vi "HB_ImaqLLGrab.vi"() -> ()   [LabVIEW 2009, in "HB_IMAQ_Examples.lvlib"]
doc: "The HL Grab VI acquires images continuously and displays the images in an image control using high-level acquisition VIs. A grab is appropriate for high-speed applications that process only one image at a time.\n\nIMAQ Init initializes the device. IMAQ Grab Setup initializes the grab function and starts capturing images to an internal software buffer. IMAQ Create creates an image buffer. IMAQ Grab Acquire copies the internal buffer to Image out, and an image control displays the image on the front panel. IMAQ Close releases resources associated with the acquisition, and IMAQ Dispose frees the image buffer."
uses:
  <vilib>/vision/driver/IMAQdx.llb/IMAQdx Buffer Number Mode.ctl
  lib.lib/HGF_LVC/HGF_IMAQ/HGF_IMAQFactory/HGF_IMAQFactory.lvclass
  lib.lib/HGF_LVC/HGF_IMAQ/HGF_IMAQDevice/HGF_IMAQDevice.lvclass
  HB_IMAQ_Examples.lvlib
  lib.lib/HGF_LVC/HGF_BaseClasses/HGF_Factory/HGF_Factory.lvclass
  lib.lib/HGF_LVC/HGF_DeviceBaseClasses/HGF_DeviceBase/HGF_DeviceBase.lvclass
  lib.lib/HGF_LVC/HGF_Auxiliary/HGF_Auxiliary.lvlib
  lib.lib/VisionTools/HGF_VisionTools/HGF_VisionTools.lvlib
  <vilib>/vision/driver/NI_Vision_Acquisition_Software.lvlib
panel:
  in  "Buffer Number Mode (Next)":T1
  out "error out":errorcluster
  in  "Number of buffers":u32=2
  out "processed FPS":dbl
  out "acquired FPS":dbl
  out "iteration":i32
  out "Image":T2(plugin-control)
  in  "interval / ms":u32=100
  in  "stop":bool
  in  "Image Type":T3 items=["Grayscale (U8)", "Grayscale (I16)", "Grayscale (SGL)", "Complex (CSG)", "RGB (U32)", "HSL (U32)", "RGB (U64)", "Grayscale (U16)"]
  in  "cameraName":string="cam0"
  in  "imaqClassName":string="HGF_ImaqDx"
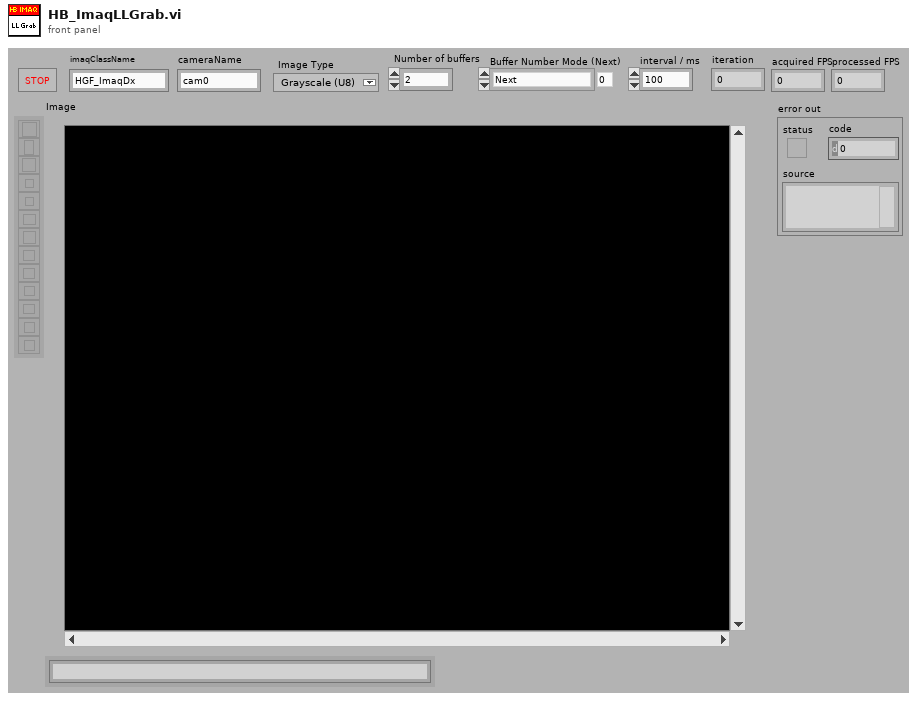
[diagram p1: front panel]
types:
  T1 = typedef "NI_Vision_Acquisition_Software.lvlib/IMAQdx Buffer Number Mode.ctl" = enum32{"Next", "Last", "Buffer Number"}
  T2 = typedef "IMAQ Image.ctl" = refnum<image>
  T3 = typedef "Image Type" = u32
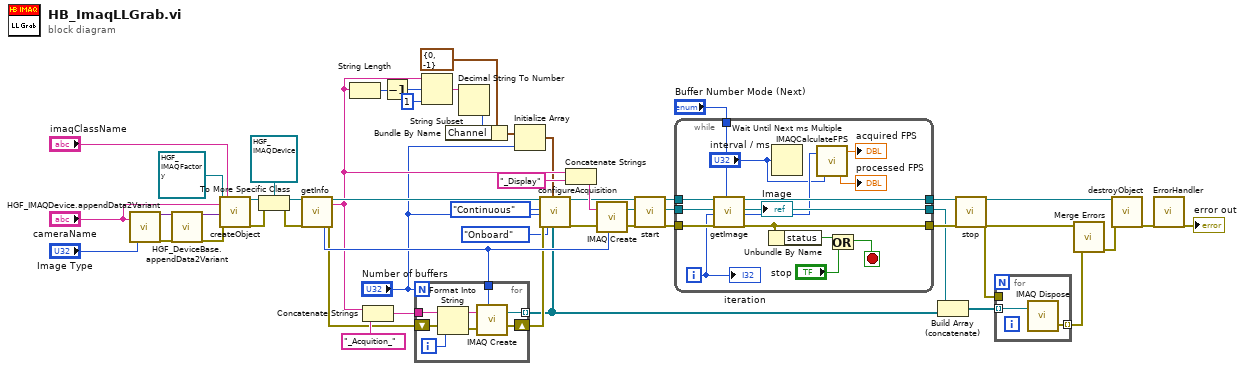
[diagram p0: block diagram]
diagram:
  n1 = call "HGF_IMAQDevice.appendData2Variant.vi"("cameraName"="cameraName", "imageType"="Image Type") -> ("dup initData"=w51:variant, "error out"=w50:errorcluster)  [unwired: 4 in, 12 out]
  n2 = call "HGF_DeviceBase.appendData2Variant.vi"("initData"=w51, "error in (no error)"=w50) -> ("dup initData"=w48:variant, "error out"=w49:errorcluster)  [unwired: 16 out]
  n3 = call "createObject.vi"("HGF_Factory"=refnum<class "HGF_IMAQFactory.lvclass"> refnum ("HGF_IMAQ.lvlib:HGF_IMAQFactory.lvclass"), "objectName"="cameraName", "initializationData"=w48, "error in (no error)"=w49, "className"="imaqClassName") -> ("HGF_Object"=w46:refnum<class "HGF_Factory.lvclass">, "error out"=w45:errorcluster)  [unwired: 13 out]
  n4 = To More Specific Class(target class=refnum<class "HGF_IMAQDevice.lvclass"> refnum ("HGF_DeviceBaseClasses.lvlib:HGF_IMAQDevice.lvclass"), reference=w46, error in=w45) -> (specific class reference=w42:refnum<class "HGF_IMAQDevice.lvclass">, error out=w41:errorcluster)
  n5 = call "getInfo.vi"("HGF_IMAQDevice"=w42, "error in (no error)"=w41) -> ("imageType"=w36:T3, "dup HGF_IMAQDevice"=w30:refnum<class "HGF_IMAQDevice.lvclass">, "cameraName"=w12:string, "error out"=w28:errorcluster)  [unwired: 12 in, 2 out]
  n6 = String Length(string=w12) -> (length=w11:i32)
  n7 = Concatenate Strings(w12, "_Acquition_" ("string")) -> (w29:string)
  n8 = Decrement(x=w11) -> (x-1=w10:i32)
  n9 = for {
    N: "Number of buffers" -> [_]
    tunnel: w36 -> [w59]
    tunnel: w29 -> [w57]
    shift-right: [w58] -> w35
    shift-left: w28 -> [w55]
    tunnel: [w52] -> w22 mode=indexing
    i -> [w53]
    n10 = Format Into String(initial string=w57, error in=w55, w53) -> (resulting string=w56:string, error out=w54:errorcluster)  [unwired: 1 in]
    n11 = call "IMAQ Create"("Image Name"=w56, "Image Type"=w59, "error in (no error)"=w54) -> ("New Image"=w52:T2, "error out"=w58:errorcluster)  [unwired: 1 in, 1 out]
  }
  n12 = String Subset(string=w12, offset (0)=w10, length (rest)=1 ("length (rest)")) -> (substring=w7:string)
  n13 = Decimal String To Number(string=w7) -> (number=w6:i32)  [unwired: 3 out]
  n14 = Bundle By Name(cluster=cluster{"Skip Count":u32, "Channel":i32} {"Skip Count"=0, "Channel"=-1} ("Buffer Parameter"), "Channel"=w6) -> (w5:cluster{"Skip Count":u32, "Channel":i32})
  n15 = Initialize Array(w5, "Number of buffers") -> (w3:cluster{"Skip Count":u32, "Channel":i32}[])
  n16 = call "configureAcquisition.vi"("HGF_IMAQDevice"=w30, "Continuous?"=enum16{"One-Shot", "Continuous"}."Continuous", "Number of buffers"="Number of buffers", "error in (no error)"=w35, "Memory Location"=enum16{"System", "Onboard"}."Onboard", "Buffer Parameters"=w3, "Image Array"=w22) -> ("dup HGF_IMAQDevice"=w27:refnum<class "HGF_IMAQDevice.lvclass">, "error out"=w34:errorcluster)  [unwired: 11 in]
  n17 = Concatenate Strings(w12, "_Display" ("string")) -> (w38:string)
  n18 = call "IMAQ Create"("Image Name"=w38, "Image Type"=w36, "error in (no error)"=w34) -> ("New Image"=w23:T2, "error out"=w25:errorcluster)  [unwired: 1 in, 1 out]
  n19 = call "start.vi"("HGF_IMAQDevice"=w27, "error in (no error)"=w25) -> ("dup HGF_IMAQDevice"=w26:refnum<class "HGF_IMAQDevice.lvclass">, "error out"=w24:errorcluster)  [unwired: 16 in]
  n20 = while {
    tunnel: w26 -> [w71]
    tunnel: w24 -> [w70]
    tunnel: w23 -> [w67]
    tunnel: [w66] -> w18
    tunnel: [w69] -> w19
    tunnel: [w68] -> w21
    tunnel: "Buffer Number Mode (Next)" -> [w64]
    i -> [w65]
    stop <- w72 stop-if-true
    n21 = call "getImage.vi"("HGF_IMAQDevice"=w71, "Image In"=w67, "Buffer Number"=w65, "error in (no error)"=w70, "Buffer Number Mode (Next)"=w64) -> ("dup HGF_IMAQDevice"=w68:refnum<class "HGF_IMAQDevice.lvclass">, "Image Out"=w66:T2, "Buffer Number Copied"=w63:i32, "error out"=w69:errorcluster)  [unwired: 8 in, 3 out]
    "Image" <- w66
    n22 = Unbundle By Name(w69) -> ("status"=w74:bool)
    n23 = Wait Until Next ms Multiple(millisecond multiple="interval / ms") -> ()  [unwired: 1 out]
    n24 = call "IMAQCalculateFPS.vi"("Update interval"="interval / ms", "buffer number"=w63) -> ("processed FPS"=→"processed FPS":dbl, "acquired FPS"=→"acquired FPS":dbl)
    n25 = Or(x=w74, y="stop") -> (x .or. y?=w72:bool)
    "iteration" <- w65
  }
  n26 = Build Array (concatenate)(w18, w22) -> (w17:T2[])
  n27 = call "stop.vi"("HGF_IMAQDevice"=w21, "error in (no error)"=w19) -> ("dup HGF_IMAQDevice"=w20:refnum<class "HGF_IMAQDevice.lvclass">, "error out"=w16:errorcluster)  [unwired: 16 in]
  n28 = for {
    tunnel: [w76] -> w15 mode=indexing
    tunnel: w16 -> [_]
    tunnel: w17 -> [w75] mode=indexing
    n29 = call "IMAQ Dispose"("Image"=w75) -> ("error out"=w76:errorcluster)  [unwired: 2 in, 3 out]
  }
  n30 = call <vilib>:"Merge Errors.vi"("error array in"=w15, "error in 1 (no error)"=w16) -> ("error out"=w14:errorcluster)  [unwired: 2 in, 3 out]
  n31 = call "destroyObject.vi"("HGF_Factory"=w20, "error in (no error)"=w14) -> ("error out"=w43:errorcluster)  [unwired: 17 out]
  n32 = call "ErrorHandler.vi"("error in (no error)"=w43) -> ("error out"=→"error out":errorcluster)  [unwired: 6 in, 12 out]
